vi "Get Project Item Type String.vi"(8 "Error In":errorcluster, 11 "ProjectItem Refnum":refnum<vi>) -> (0 "Error Out":errorcluster, 2 "Type String":string, 3 "ProjectItem Refnum Out":refnum<vi>)   [LabVIEW 2014, in "i3-docs.lvlib"]
uses:
  i3-docs.lvlib
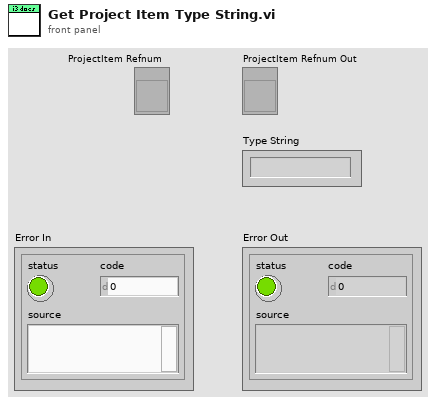
[diagram p1: front panel]
types:
  T1 = enum32{"invalid VI type", "Standard VI", "Control VI", "Global VI", "Polymorphic VI", "Configuration VI", "SubSystem", "Facade VI", "Method VI", "Statechart Diagram VI"}
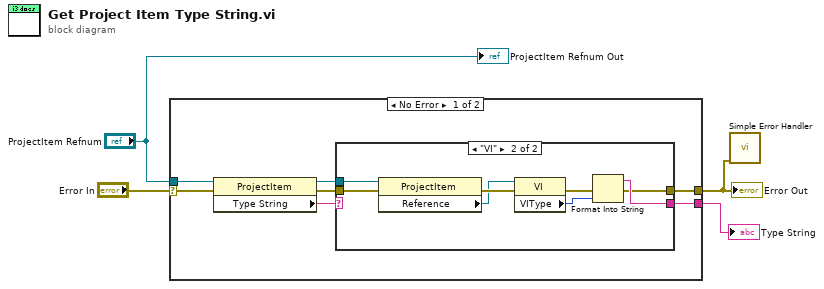
[diagram p0: block diagram]
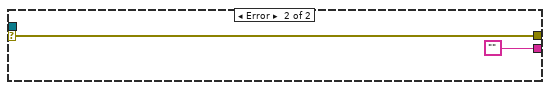
[diagram p3: hidden frame]
diagram:
  n1 = case shown="No Error" "Error In" {
    selector: "Error In" -> [w7 w22]
    tunnel: "ProjectItem Refnum" -> [w11 _]
    tunnel: [w8 ""] -> w4
    tunnel: [w5 w22] -> w1
    frame No Error {
      n2 = property class="ProjectItem"(reference=w11, error in=w7) -> (reference out=w9:refnum<vi>, error out=w6:errorcluster, "Type String"=w10:string)
      n3 = case shown="\"VI\"" w10 {
        selector: w10 -> [w13 _]
        tunnel: w9 -> [_ w21]
        tunnel: [w13 w15] -> w8
        tunnel: w6 -> [w12 w20]
        tunnel: [w12 w14] -> w5
        frame Default {
        }
        frame "VI" {
          n4 = property class="ProjectItem"(reference=w21, error in=w20) -> (error out=w19:errorcluster, "Reference"=w18:refnum<vi>)  [unwired: 1 out]
          n5 = property class="VI"(reference=w18, error in=w19) -> (error out=w16:errorcluster, "VIType"=w17:T1)  [unwired: 1 out]
          n6 = Format Into String(error in=w16, w17) -> (resulting string=w15:string, error out=w14:errorcluster)  [unwired: 2 in]
        }
      }
    }
    frame Error {
    }
  }
  "Error Out" <- w1
  "Type String" <- w4
  n7 = call <vilib>:"Simple Error Handler.vi"("error in (no error)"=w1) -> ()  [unwired: 4 in, 5 out]
  "ProjectItem Refnum Out" <- "ProjectItem Refnum"
